vi "scale (SubVI).vi"(4 "data":i32) -> (1 "output":i8)   [LabVIEW 2013]
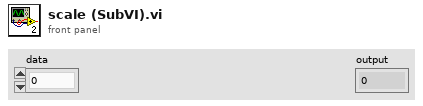
[diagram p1: front panel]
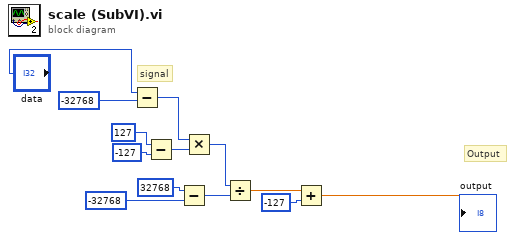
[diagram p0: block diagram]
diagram:
  # "Output"
  # "signal"
  n1 = Subtract(x="data", y=-32768) -> (x-y=w6:i32)
  n2 = Subtract(x=127, y=-127) -> (x-y=w7:i32)
  n3 = Subtract(x=32768, y=-32768) -> (x-y=w8:i32)
  n4 = Multiply(x=w6, y=w7) -> (x*y=w5:i32)
  n5 = Divide(x=w5, y=w8) -> (x/y=w4:dbl)
  n6 = Add(x=w4, y=-127) -> (x+y=→"output":dbl)
